vi "GetGas.vi"(7 "Timeout (ms)":u32=2000, 8 "Error In":errorcluster, 11 "Sierra M100 In":refnum<visa-resource-name>) -> (0 "Error Out":errorcluster, 2 "Gas":T1, 3 "Sierra M100 Out":refnum<visa-resource-name>)   [LabVIEW 2012, in "Sierra-M100.lvlib"]
doc: "This VI gets the has currently used with the mass flow controller."
uses:
  Sierra-M100.lvlib
  Controls/Gas.ctl
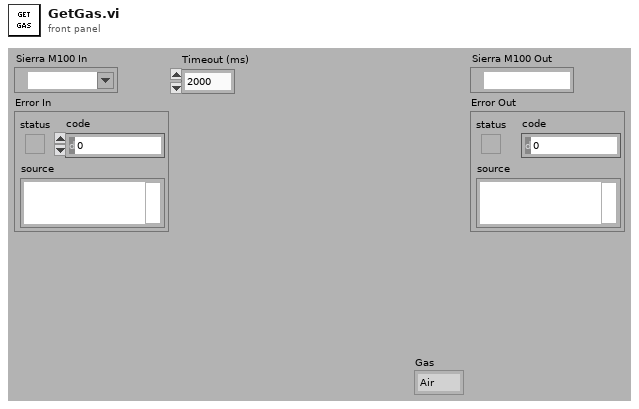
[diagram p1: front panel]
types:
  T1 = typedef "Sierra-M100.lvlib/Gas.ctl" = enum16{"Air", "Argon", "CO2", "CO", "Helium", "Hydrogen", "Methane", "Nitrogen", "Nitrous Oxide", "Oxygen"}
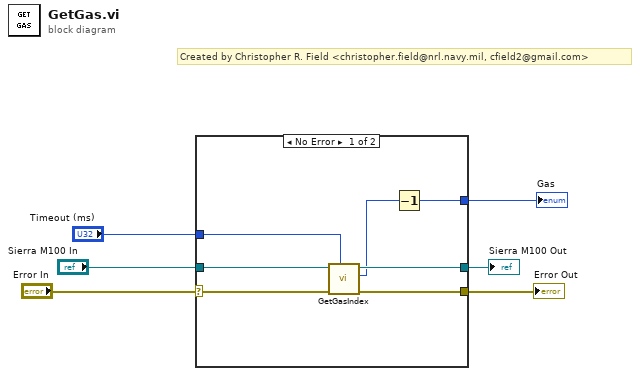
[diagram p0: block diagram]
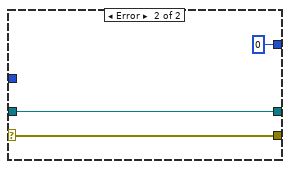
[diagram p2: hidden frame]
diagram:
  # "Created by Christopher R. Field <christopher.field@nrl.navy.mil, cfield2@gmail.com>"
  n1 = case shown="No Error" "Error In" {
    selector: "Error In" -> [w7 w15]
    tunnel: "Sierra M100 In" -> [w13 w16]
    tunnel: [w12 w16] -> w5
    tunnel: [w11 w15] -> w4
    tunnel: [w9 u16 0] -> w3
    tunnel: "Timeout (ms)" -> [w8 _]
    frame No Error {
      n2 = call "GetGasIndex.vi"("Timeout (ms)"=w8, "Error In"=w7, "Sierra M100 In"=w13) -> ("Error Out"=w11:errorcluster, "Gas Index"=w10:u16, "Sierra M100 Out"=w12:refnum<visa-resource-name>)  [unwired: 6 in]
      n3 = Decrement(x=w10) -> (x-1=w9:u16)
    }
    frame Error {
    }
  }
  "Sierra M100 Out" <- w5
  "Error Out" <- w4
  "Gas" <- w3
